vi "HRM-Stage5-GUI_main.vi"(8 "error in (no error)":errorcluster, 11 "Init cluster":T1) -> (0 "error out":errorcluster)   [LabVIEW 2020]
uses:
  Stage 4/initclose/HRM-Stage4-init_cluster.ctl
  Stage 4/initclose/HRM-stage4-config_data.ctl
  Stage 4/initclose/HRM-Stage4-User_events.ctl
  Stage 4/process/HRM-process-peak_detect_setting.ctl
panel:
  in  "Tab Control":enum32{"Filtered", "unfiltered wf"}(tab)
  out "Filtered":waveform(dbl)(graph)
  out "unfiltered wf":waveform(dbl)(graph)
  in  "Top":dbl
  in  "Bot":dbl
  in  "Peak Detection":bool
  in  "Clear data":bool
  in  "Run Aquisition?":bool
  out "Feedback":string
  out "Pulse":dbl
  in  "Addition signal to remove (0) [s]":dbl
  in  "Samples size (10) [s]":i32=10
  in  "Stop":bool
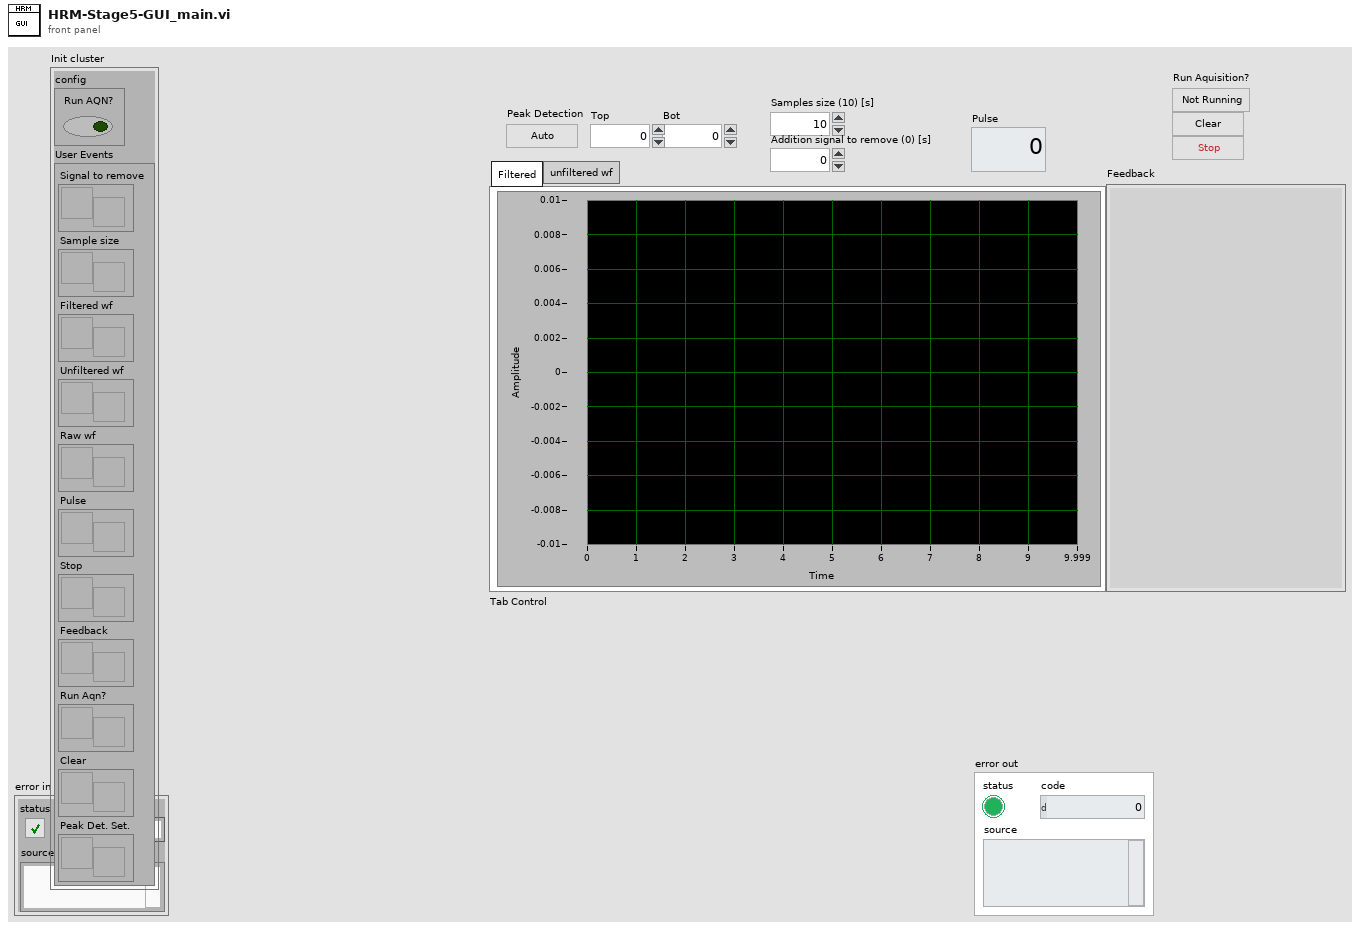
[diagram p1: front panel]
types:
  T1 = typedef "HRM-Stage4-init_cluster.ctl" = cluster{"config":T2, "User Events":T3}
  T2 = typedef "HRM-stage4-config_data.ctl" = cluster{"Run AQN?":bool}
  T3 = typedef "HRM-Stage4-User_events.ctl" = cluster{"Signal to remove":refnum<user-event>, "Sample size":refnum<user-event>, "Filtered wf":refnum<user-event>, "Unfiltered wf":refnum<user-event>, "Raw wf":refnum<user-event>, "Pulse":refnum<user-event>, "Stop":refnum<user-event>, "Feedback":refnum<user-event>, "Run Aqn?":refnum<user-event>, "Clear":refnum<user-event>, "Peak Det. Set.":refnum<user-event>}
  T4 = typedef "HRM-process-peak_detect_setting.ctl" = cluster{"Manual?":bool, "Top":dbl, "Bot":dbl}
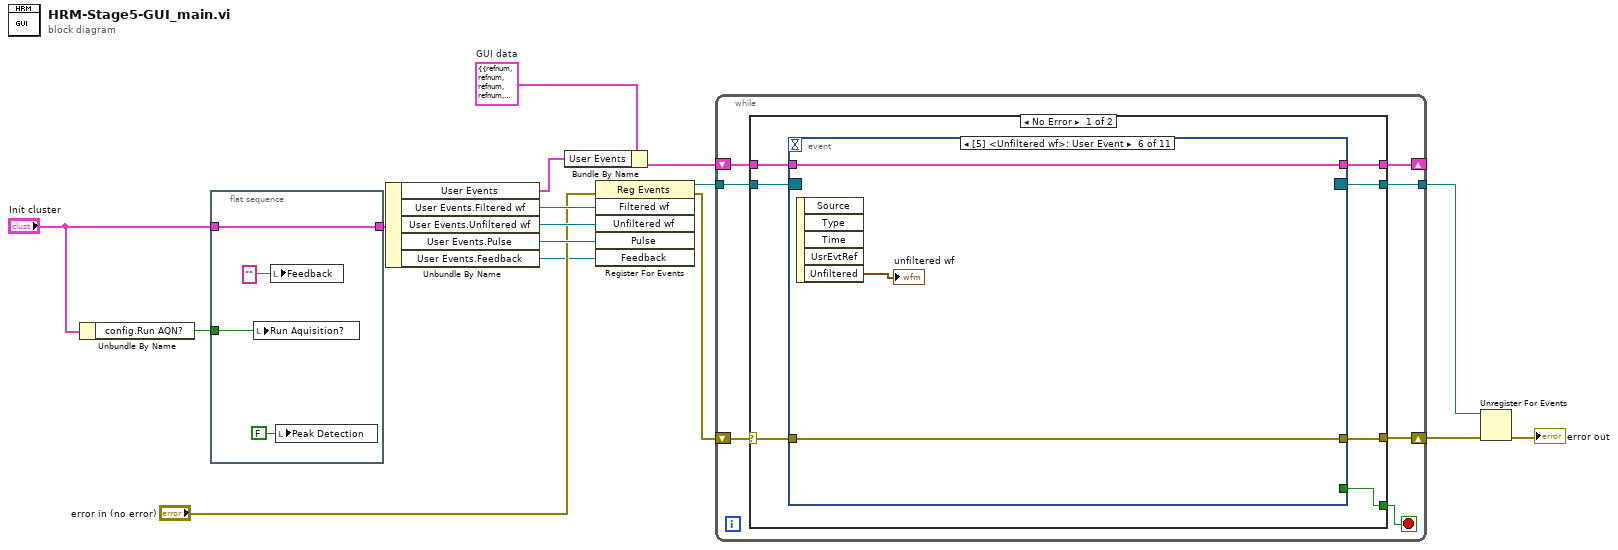
[diagram p0: block diagram]
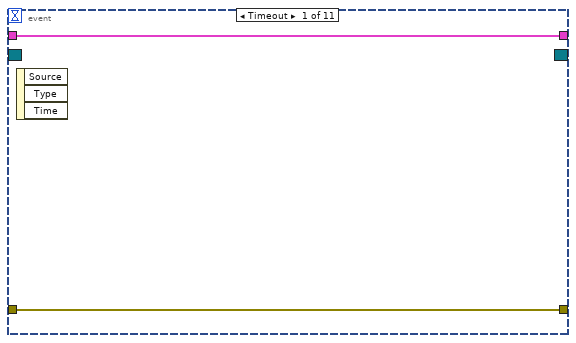
[diagram p2: hidden frame]
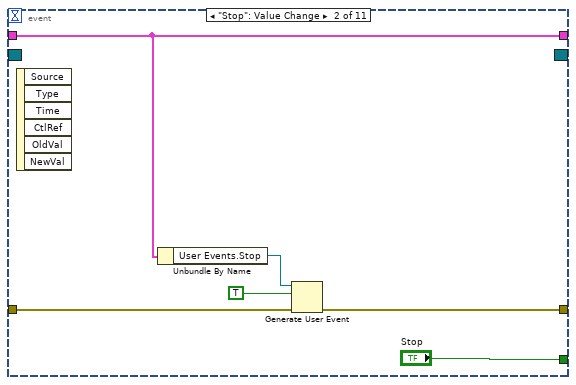
[diagram p3: hidden frame]
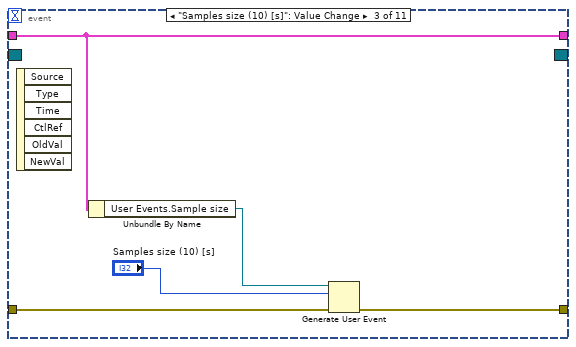
[diagram p4: hidden frame]
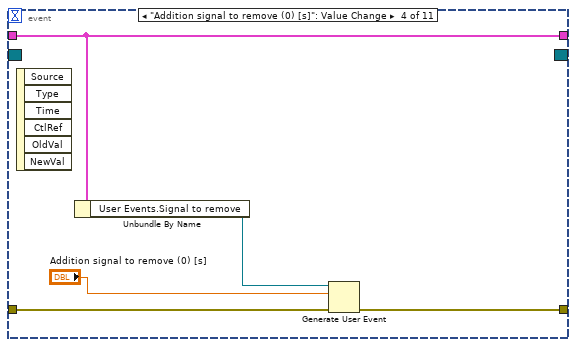
[diagram p5: hidden frame]
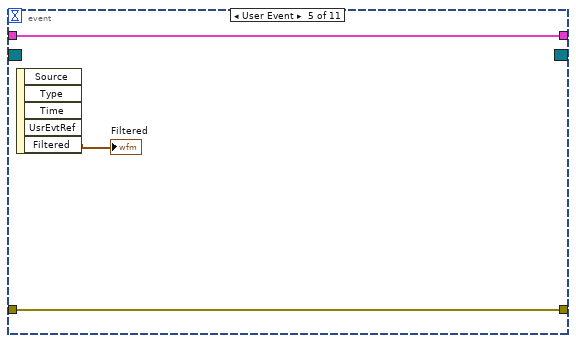
[diagram p6: hidden frame]
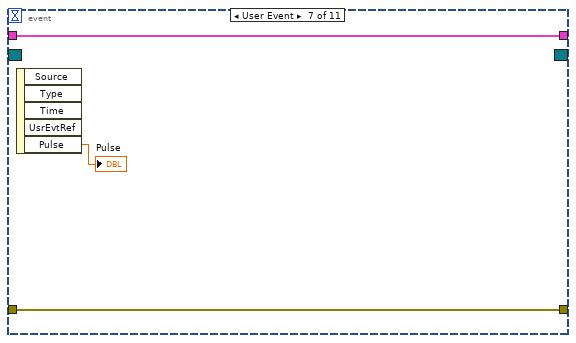
[diagram p7: hidden frame]
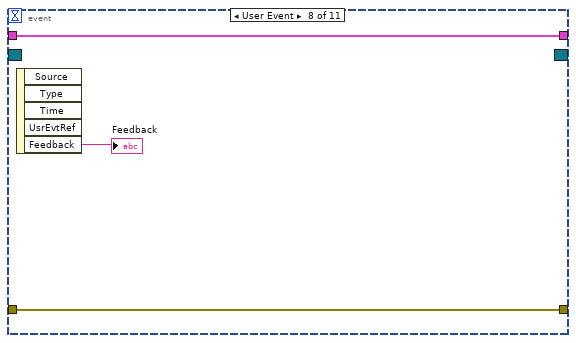
[diagram p8: hidden frame]
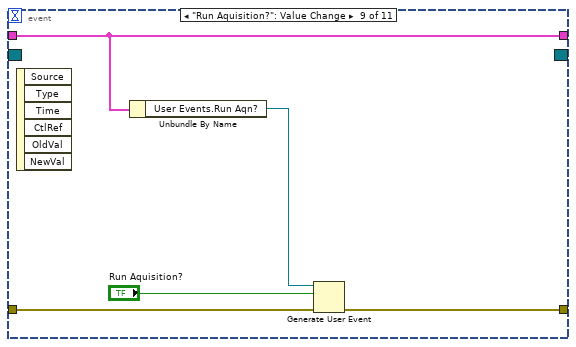
[diagram p9: hidden frame]
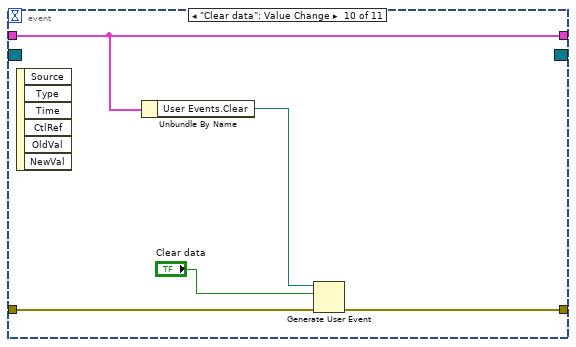
[diagram p10: hidden frame]
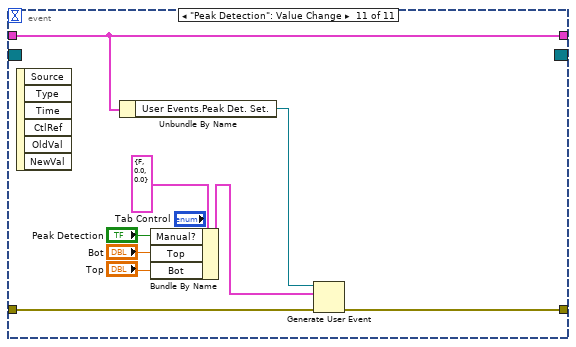
[diagram p11: hidden frame]
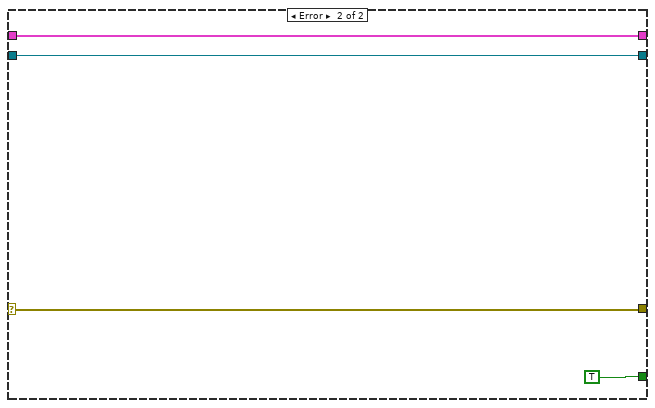
[diagram p12: hidden frame]
diagram:
  w15 = cluster{"User Events":T3} {"User Events"={"Signal to remove"=refnum, "Sample size"=refnum, "Filtered wf"=refnum, "Unfiltered wf"=refnum, "Raw wf"=refnum, "Pulse"=refnum, "Stop"=refnum, "Feedback"=refnum, "Run Aqn?"=refnum, "Clear"=refnum, "Peak Det. Set."=refnum}}  # GUI data
  n1 = Unbundle By Name("Init cluster") -> ("config.Run AQN?"=w1:bool)
  n2 = flat-sequence {
    tunnel: "Init cluster" -> [w20]
    tunnel: [w20] -> w3
    tunnel: w1 -> [w18]
    frame #0 {
      n3 = local write "Run Aquisition?"(w18) -> ()
      n4 = local write "Feedback"("") -> ()
      n5 = local write "Peak Detection"(FALSE ("Peak Detection")) -> ()
    }
  }
  n6 = Unbundle By Name(w3) -> ("User Events"=w10:T3, "User Events.Filtered wf"=w9:refnum<user-event>, "User Events.Unfiltered wf"=w8:refnum<user-event>, "User Events.Pulse"=w7:refnum<user-event>, "User Events.Feedback"=w4:refnum<user-event>)
  n7 = Bundle By Name(cluster=w15, "User Events"=w10) -> (w11:cluster{"User Events":T3})
  n8 = register-events(error in="error in (no error)", w9, w8, w7, w4) -> (reference out=w16:refnum<event-registration>, error out=w14:errorcluster)  [unwired: 1 in]
  n9 = while {
    tunnel: w16 -> [w27]
    shift-right: [w23] -> w12
    shift-left: w14 -> [w24]
    shift-right: [w22] -> _
    shift-left: w11 -> [w26]
    tunnel: [w21] -> w13
    stop <- w25 stop-if-true
    n10 = case shown="No Error" w24 {
      selector: w24 -> [w31 w86]
      tunnel: [w32 TRUE ("Stop")] -> w25
      tunnel: [w30 w86] -> w23
      tunnel: w27 -> [w34 w84]
      tunnel: w26 -> [w33 w85]
      tunnel: [w29 w85] -> w22
      tunnel: [w28 w84] -> w21
      frame No Error {
        n11 = event shown="[5] <Unfiltered wf>: User Event" {
          selector: w34 -> [_ _ _ _ _ _ _ _ _ _ _]
          dyn-events: [_ _ _ _ _ _ _ _ _ _ _] -> w28
          timeout: _ -> [_ _ _ _ _ _ _ _ _ _ _]
          tunnel: w33 -> [w36 w41 w45 w50 w54 w57 w60 w63 w69 w74 w83]
          tunnel: [_ "Stop" _ _ _ _ _ _ _ _ _] -> w32
          tunnel: [w35 w38 w46 w51 w55 w58 w61 w64 w66 w71 w80] -> w30
          tunnel: w31 -> [w35 w39 w47 w52 w55 w58 w61 w64 w67 w72 w81]
          tunnel: [w36 w41 w45 w50 w54 w57 w60 w63 w69 w74 w83] -> w29
          event Timeout {
            n12 = event-data() -> ()  [unwired: 1 in, 3 out]
          }
          event "Stop": Value Change {
            n13 = event-data() -> ()  [unwired: 1 in, 6 out]
            n14 = Unbundle By Name(w41) -> ("User Events.Stop"=w40:refnum<user-event>)
            n15 = Generate User Event(user event=w40, event data cluster=TRUE ("event data"), error in=w39) -> (error out=w38:errorcluster)  [unwired: 1 in, 1 out]
          }
          event "Samples size (10) [s]": Value Change {
            n16 = event-data() -> ()  [unwired: 1 in, 6 out]
            n17 = Unbundle By Name(w45) -> ("User Events.Sample size"=w44:refnum<user-event>)
            n18 = Generate User Event(user event=w44, event data cluster="Samples size (10) [s]", error in=w47) -> (error out=w46:errorcluster)  [unwired: 1 in, 1 out]
          }
          event "Addition signal to remove (0) [s]": Value Change {
            n19 = event-data() -> ()  [unwired: 1 in, 6 out]
            n20 = Unbundle By Name(w50) -> ("User Events.Signal to remove"=w49:refnum<user-event>)
            n21 = Generate User Event(user event=w49, event data cluster="Addition signal to remove (0) [s]", error in=w52) -> (error out=w51:errorcluster)  [unwired: 1 in, 1 out]
          }
          event User Event {
            n22 = event-data() -> ("Filtered"=→"Filtered":waveform(dbl))  [unwired: 1 in, 4 out]
          }
          event User Event {
            n23 = event-data() -> ("Unfiltered"=→"unfiltered wf":waveform(dbl))  [unwired: 1 in, 4 out]
          }
          event User Event {
            n24 = event-data() -> ("Pulse"=→"Pulse":dbl)  [unwired: 1 in, 4 out]
          }
          event User Event {
            n25 = event-data() -> ("Feedback"=→"Feedback":string)  [unwired: 1 in, 4 out]
          }
          event "Run Aquisition?": Value Change {
            n26 = event-data() -> ()  [unwired: 1 in, 6 out]
            n27 = Unbundle By Name(w69) -> ("User Events.Run Aqn?"=w68:refnum<user-event>)
            n28 = Generate User Event(user event=w68, event data cluster="Run Aquisition?", error in=w67) -> (error out=w66:errorcluster)  [unwired: 1 in, 1 out]
          }
          event "Clear data": Value Change {
            n29 = event-data() -> ()  [unwired: 1 in, 6 out]
            n30 = Unbundle By Name(w74) -> ("User Events.Clear"=w73:refnum<user-event>)
            n31 = Generate User Event(user event=w73, event data cluster="Clear data", error in=w72) -> (error out=w71:errorcluster)  [unwired: 1 in, 1 out]
          }
          event "Peak Detection": Value Change {
            n32 = event-data() -> ()  [unwired: 1 in, 6 out]
            n33 = Unbundle By Name(w83) -> ("User Events.Peak Det. Set."=w82:refnum<user-event>)
            n34 = Bundle By Name(cluster=T4 {"Manual?"=FALSE, "Top"=0.0, "Bot"=0.0} ("event data"), "Manual?"="Peak Detection", "Top"="Bot", "Bot"="Top") -> (w78:T4)
            n35 = Generate User Event(user event=w82, event data cluster=w78, error in=w81) -> (error out=w80:errorcluster)  [unwired: 1 in, 1 out]
          }
        }
      }
      frame Error {
      }
    }
  }
  n36 = Unregister For Events(event registration refnum=w13, error in=w12) -> (error out=→"error out":errorcluster)
